vi "SV TDMS Read Spectrum (Colormap).vi"(0 "tdms file":refnum<k34>, 5 "group name in":string="Colormap", 11 "error in":errorcluster) -> (3 "scale labels":T1, 4 "tdms file out":refnum<k34>, 6 "group name out":string="Colormap", 10 "colormap":T8, 13 "spectrum info":T2 {"x-axis units" items=["Time (s)"=0, "Frequency-CB (Hz)"=1, "Frequency-CPB (Hz)"=1248, "Frequency-Arbitrary (Hz)"=2357, "Quefrency (s)"=2, "Revolutions (rev)"=3, "Order"=4, "Speed (RPM)"=11, "Speed (rad/s)"=21, "Index"=65535]; "weighting filter" items=["Linear", "A-weighting", "B-weighting", "C-weighting", "ITU-R 468-4", "Dolby", "CCITT", "C-message", "Wb", "Wc", "Wd", "We", "Wf", "Wh", "Wj", "Wk", "Wm", "AES17 20 kHz lowpass", "AES17 40 kHz lowpass", "AES17 20 kHz highpass", "AES17 40 kHz highpass"]; "dB reference [EU]" format="%.2f"; "engineering units" items=["custom..."=0, "V"=1, "A"=21, "C"=30, "pC"=31, "s"=32, "-"=29, "Pa"=2, "N"=20, "g"=3, "m/s^2"=4, "m/s"=5, "m"=6, "mm/s"=12, "mm"=13, "micron/s"=14, "micron"=15, "in/s^2"=7, "in/s"=8, "in"=9, "mil/s"=10, "mil"=11, "rad/s^2"=16, "rad/s"=17, "rad"=18, "deg/s^2"=26, "deg/s"=27, "deg"=28, "RPM"=22, "cycle/s^2"=23, "Hz"=24, "cycle"=25, "strain"=19]; "spectral info"."window" items=["None "=0, "Hanning"=1, "Hamming"=2, "Blackman-Harris"=3, "Exact Blackman"=4, "Blackman"=5, "Flat Top"=6, "4 Term B-Harris "=7, "7 Term B-Harris"=8, "Low Sidelobe"=9, "Force - Exponential"=10, "Gaussian"=62]}, 15 "error out":errorcluster)   [LabVIEW 2017]
doc: "Reads the specified .tdms file and returns data in a format specific to the polymorphic instance selected."
uses:
  <vilib>/addons/_NISVFA/_Shared subVIs/Controls/svc_Spectrum Info.ctl
  <vilib>/addons/_NISVFA/_Shared subVIs/Controls/svc_X-Axis Units.ctl
  <vilib>/addons/_NISVFA/_Shared subVIs/Controls/svc_Spectrum Type.ctl
  <vilib>/addons/_NISVFA/_Shared subVIs/Controls/svc_Engineering Units Text Ring.ctl
  <vilib>/addons/_NISVFA/_Shared subVIs/Controls/svc_Weighting Filter Text Ring.ctl
  <vilib>/addons/_NISVFA/_Shared subVIs/Controls/svc_Complimentary Spectrum Units.ctl
  <vilib>/addons/_NISVFA/_Shared subVIs/Controls/NI Spectrum Component.ctl
  <vilib>/addons/_NISVFA/_Shared subVIs/Controls/svc_Speed Profile.ctl
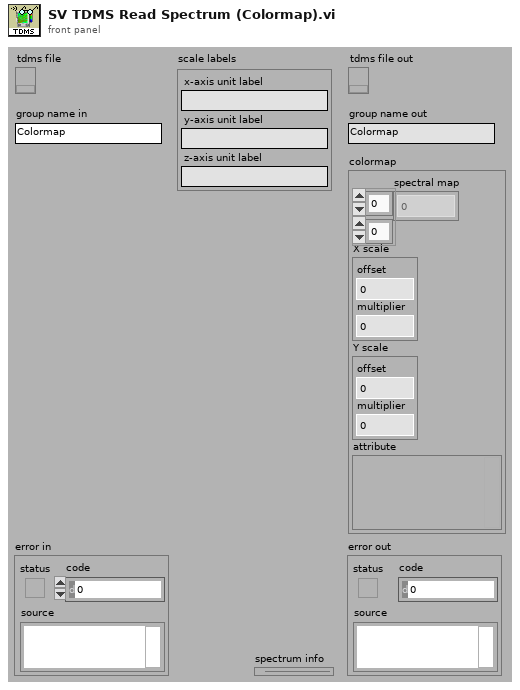
[diagram p1: front panel]
types:
  T1 = cluster{"x-axis unit label":string, "y-axis unit label":string, "z-axis unit label":string}
  T2 = typedef "svc_Spectrum Info.ctl" = cluster{"channel name":string, "description":string, "x-axis units":T3, "spectral info":cluster{"spectrum type":T4, "linear/dB":enum16{"linear", "dB"}, "window":u16, "window size":i32, "FFT size":i32}, "engineering units":T5, "custom label":string, "dB reference [EU]":dbl, "peak units":enum16{"rms", "peak", "peak-peak"}, "weighting filter":T6, "spectral density?":bool, "unit label":string, "spectrum skewed?":bool, "complimentary spectrum units":T7}
  T3 = typedef "svc_X-Axis Units.ctl" = u16
  T4 = typedef "svc_Spectrum Type.ctl" = enum16{"FFT Spectrum [complex]", "Amplitude [Magnitude]", "Power [Magnitude^2]", "Cross Spectrum [complex]", "Frequency Response [Complex]"}
  T5 = typedef "svc_Engineering Units Text Ring.ctl" = u16
  T6 = typedef "svc_Weighting Filter Text Ring.ctl" = u16
  T7 = typedef "svc_Complimentary Spectrum Units.ctl" = enum16{"none", "radians", "degrees", "cycles", "imaginary"}
  T8 = cluster{"spectral map":dbl[][], "X scale":cluster{"offset":dbl, "multiplier":dbl}, "Y scale":cluster{"offset":dbl, "multiplier":dbl}, "attribute":variant}
  T9 = typedef "NI Spectrum Component.ctl" = u16
  T10 = enum16{"Frequency-Time", "Time-Frequency", "Order-Time", "Time-Order", "Frequency-RPM", "RPM-Frequency", "Order-RPM", "RPM-Order"}
  T11 = typedef "svc_Speed Profile.ctl" = cluster{"time [s]":dbl[], "speed [RPM]":dbl[]}
  T12 = cluster{"name":string, "name":string, "scale label with units":string}
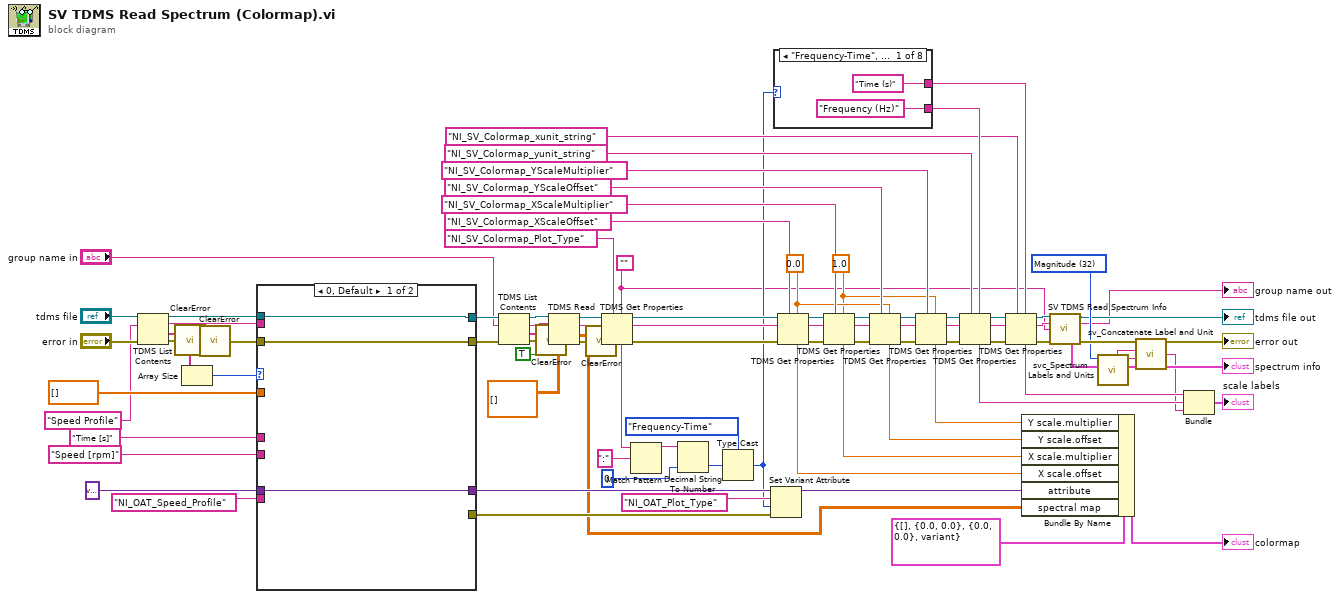
[diagram p0: block diagram]
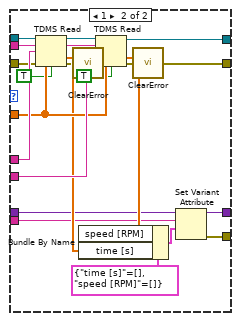
[diagram p2: hidden frame]
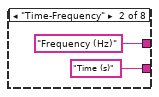
[diagram p3: hidden frame]
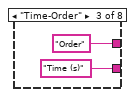
[diagram p4: hidden frame]
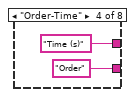
[diagram p5: hidden frame]
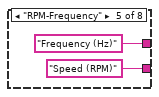
[diagram p6: hidden frame]
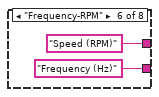
[diagram p7: hidden frame]
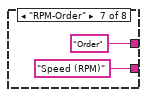
[diagram p8: hidden frame]
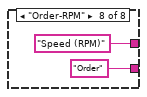
[diagram p9: hidden frame]
diagram:
  w23 = T9 32 items=["Magnitude"=32, "Phase"=33, "Real"=34, "Imaginary"=35, "Coherence"=36, "Unknown"=99] ("spectrum component")
  w37 = 1.0 ("X scale.multiplier")
  w38 = 0.0 ("X scale.multiplier")
  w11 = "" ("property values")
  n1 = TDMS List Contents(4:"error in", 6:"Speed Profile" ("name"), 7:"tdms file") -> (0:w2:errorcluster, 1:w7:string[], 2:w13:string, 3:w15:refnum<k34>)
  n2 = call <vilib>:"ClearError.vi"("error in (no error)"=w2) -> ("error out"=w4:errorcluster)
  n3 = Array Size(array=w7) -> (size(s)=w12:i32)
  n4 = call <vilib>:"ClearError.vi"("error in (no error)"=w4) -> ("error out"=w3:errorcluster)
  n5 = case shown="0, Default" w12 {
    tunnel: [w94 w118] -> w86
    tunnel: [w95 w117] -> w85
    tunnel: "Time [s]" ("name") -> [_ w115]
    tunnel: "Speed [rpm]" ("name") -> [_ w114]
    tunnel: dbl[] [] ("speed [RPM]") -> [_ w111]
    tunnel: variant ("variant") -> [w93 w107]
    tunnel: [w93 w106] -> w48
    tunnel: [_ w105] -> w47
    tunnel: "NI_OAT_Speed_Profile" ("name") -> [_ w104]
    tunnel: w3 -> [w94 w103]
    tunnel: w15 -> [w95 w102]
    tunnel: w13 -> [_ w101]
    frame 0, Default {
    }
    frame 1 {
      n6 = TDMS Read(0:w102, 5:w101, 7:w115, 11:w103, 12:w111, 13:TRUE ("return channels in file order? (F)")) -> (4:w116:refnum<k34>, 6:w113:string, 10:w109:dbl[], 15:w98:errorcluster)  [unwired: 2 in, 2 out]
      n7 = call <vilib>:"ClearError.vi"("error in (no error)"=w98) -> ("error out"=w112:errorcluster)
      n8 = TDMS Read(0:w116, 5:w113, 7:w114, 11:w112, 12:w111, 13:TRUE ("return channels in file order? (F)")) -> (4:w117:refnum<k34>, 10:w108:dbl[], 15:w99:errorcluster)  [unwired: 2 in, 3 out]
      n9 = Bundle By Name(cluster=T11 {"time [s]"=[], "speed [RPM]"=[]} ("speed profile"), "speed [RPM]"=w108, "time [s]"=w109) -> (w100:T11)
      n10 = call <vilib>:"ClearError.vi"("error in (no error)"=w99) -> ("error out"=w118:errorcluster)
      n11 = Set Variant Attribute(Variant=w107, name=w104, value=w100) -> (Variant out=w106:variant, error out=w105:errorcluster)  [unwired: 1 in, 1 out]
    }
  }
  n12 = TDMS List Contents(4:w86, 6:"group name in", 7:w85) -> (0:w1:errorcluster, 1:w6:string[], 2:w5:string, 3:w84:refnum<k34>)
  n13 = call <vilib>:"ClearError.vi"("error in (no error)"=w1) -> ("error out"=w60:errorcluster)
  n14 = TDMS Read(0:w84, 5:w5, 7:w6, 11:w60, 12:dbl[][] [] ("data"), 13:TRUE ("return channels in file order? (F)")) -> (4:w59:refnum<k34>, 6:w58:string, 10:w34:dbl[][], 15:w9:errorcluster)  [unwired: 2 in, 2 out]
  n15 = call <vilib>:"ClearError.vi"("error in (no error)"=w9) -> ("error out"=w56:errorcluster)
  n16 = TDMS Get Properties(5:w11, 7:"NI_SV_Colormap_Plot_Type" ("name"), 8:w56, 10:w58, 11:w59) -> (0:w82:errorcluster, 2:w81:string, 3:w83:refnum<k34>, 4:w45:string)  [unwired: 1 in, 2 out]
  n17 = Match Pattern(string=w45, regular expression=":") -> (before substring=w46:string)  [unwired: 1 in, 3 out]
  n18 = Decimal String To Number(string=w46, default (0L)=u16 0 ("default (0 I32)")) -> (number=w43:u16)  [unwired: 1 in, 1 out]
  n19 = Type Cast(type=T10."Frequency-Time" ("plot type"), x=w43) -> (*(type *) &x=w36:T10)
  n20 = Set Variant Attribute(Variant=w48, name="NI_OAT_Plot_Type", value=w36, error in=w47) -> (Variant out=w40:variant)  [unwired: 2 out]
  n21 = case shown="\"Frequency-Time\", Default" w36 {
    tunnel: ["Time (s)" ("name") "Frequency (Hz)" ("name") "Order" ("name") "Time (s)" ("name") "Frequency (Hz)" ("name") "Speed (RPM)" ("name") "Order" ("name") "Speed (RPM)" ("name")] -> w88
    tunnel: ["Frequency (Hz)" ("name") "Time (s)" ("name") "Time (s)" ("name") "Order" ("name") "Speed (RPM)" ("name") "Frequency (Hz)" ("name") "Speed (RPM)" ("name") "Order" ("name")] -> w89
    frame "Frequency-Time", Default {
    }
    frame "Time-Frequency" {
    }
    frame "Time-Order" {
    }
    frame "Order-Time" {
    }
    frame "RPM-Frequency" {
    }
    frame "Frequency-RPM" {
    }
    frame "RPM-Order" {
    }
    frame "Order-RPM" {
    }
  }
  n22 = TDMS Get Properties(5:w38, 7:"NI_SV_Colormap_XScaleOffset" ("channel name"), 8:w82, 10:w81, 11:w83) -> (0:w63:errorcluster, 2:w64:string, 3:w65:refnum<k34>, 4:w35:dbl)  [unwired: 1 in, 2 out]
  n23 = TDMS Get Properties(5:w37, 7:"NI_SV_Colormap_XScaleMultiplier" ("channel name"), 8:w63, 10:w64, 11:w65) -> (0:w80:errorcluster, 2:w70:string, 3:w69:refnum<k34>, 4:w33:dbl)  [unwired: 1 in, 2 out]
  n24 = TDMS Get Properties(5:w38, 7:"NI_SV_Colormap_YScaleOffset" ("channel name"), 8:w80, 10:w70, 11:w69) -> (0:w68:errorcluster, 2:w67:string, 3:w66:refnum<k34>, 4:w32:dbl)  [unwired: 1 in, 2 out]
  n25 = TDMS Get Properties(5:w37, 7:"NI_SV_Colormap_YScaleMultiplier" ("channel name"), 8:w68, 10:w67, 11:w66) -> (0:w92:errorcluster, 2:w91:string, 3:w90:refnum<k34>, 4:w31:dbl)  [unwired: 1 in, 2 out]
  n26 = TDMS Get Properties(5:w89, 7:"NI_SV_Colormap_yunit_string" ("channel name"), 8:w92, 10:w91, 11:w90) -> (0:w75:errorcluster, 2:w76:string, 3:w77:refnum<k34>, 4:w26:string)  [unwired: 1 in, 2 out]
  n27 = TDMS Get Properties(5:w88, 7:"NI_SV_Colormap_xunit_string" ("channel name"), 8:w75, 10:w76, 11:w77) -> (0:w30:errorcluster, 2:w29:string, 3:w28:refnum<k34>, 4:w27:string)  [unwired: 1 in, 2 out]
  n28 = Bundle By Name(cluster=T8 {"spectral map"=[], "X scale"={"offset"=0.0, "multiplier"=0.0}, "Y scale"={"offset"=0.0, "multiplier"=0.0}, "attribute"=variant} ("input cluster"), "Y scale.multiplier"=w31, "Y scale.offset"=w32, "X scale.multiplier"=w33, "X scale.offset"=w35, "attribute"=w40, "spectral map"=w34) -> (→"colormap":T8)
  n29 = call <vilib>:"SV TDMS Read Spectrum Info.vi"("tdms file"=w28, "group name in"=w29, "channel name in"=w11, "error in"=w30) -> ("tdms file out"=→"tdms file out":refnum<k34>, "group name out"=→"group name out":string, "spectrum info"=w25:T2, "error out"=→"error out":errorcluster)  [unwired: 7 in, 1 out]
  n30 = call <vilib>:"svc_Spectrum Labels and Units.vi"("spectrum info in"=w25, "spectrum component"=w23) -> ("spectrum info out"=→"spectrum info":T2, "unit label"=w22:string, "y-axis label"=w21:string)  [unwired: 4 in, 3 out]
  n31 = call <vilib>:"sv_Concatenate Label and Unit.vi"("unit string"=w22, "label"=w21) -> ("scale label with units"=w20:string)  [unwired: 4 in]
  n32 = Bundle("name"=w27, "name"=w26, "scale label with units"=w20) -> (→"scale labels":T12)  [unwired: 1 in]
